vi "Test Runner Pre-build action.vi"(6 "Top Level/Always Included VIs":path[](array[path]), 7 "Main Destination Path":path, 9 "Target Name":string, 10 "Build Specification Name":string, 11 "Project Path":path) -> (0 "error out":errorcluster)   [LabVIEW 2013]
uses:
  classes/Test Runner/Test Runner.lvclass
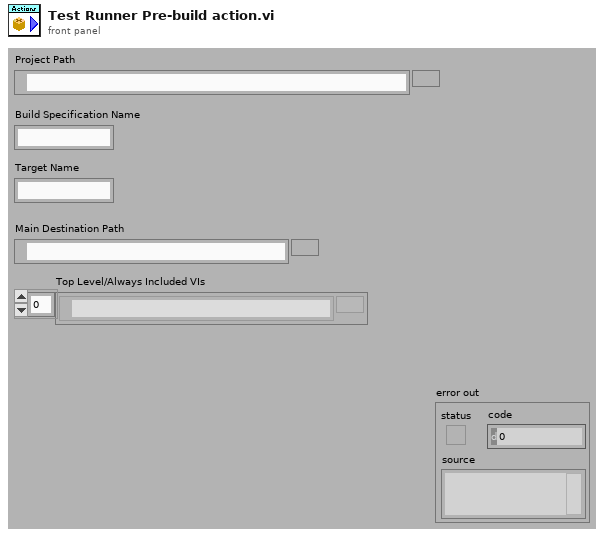
[diagram p1: front panel]
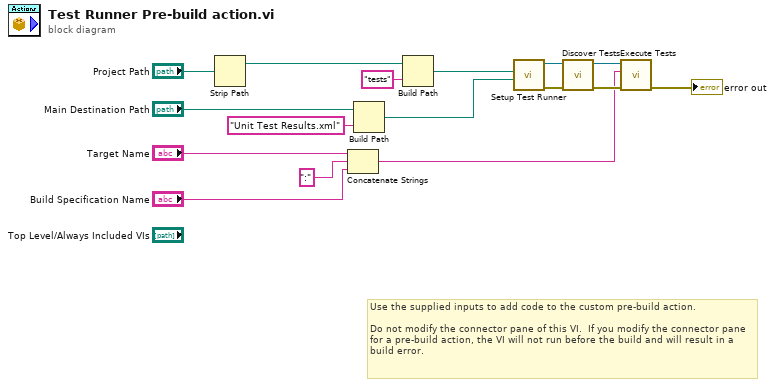
[diagram p0: block diagram]
diagram:
  # "Use the supplied inputs to add code to the custom pre-build action.\n\nDo not modify the connector pane of this VI.  If you modify the connector pane for a pre-build action, the VI will not run before the build and will result in a build error."
  n1 = Strip Path(path="Project Path") -> (stripped path=w1:path)  [unwired: 1 out]
  n2 = Concatenate Strings("Target Name", ":" ("string"), "Build Specification Name") -> (w6:string)
  n3 = Build Path(base path="Main Destination Path", name or relative path="Unit Test Results.xml") -> (appended path=w2:path)
  n4 = Build Path(base path=w1, name or relative path="tests") -> (appended path=w4:path)
  n5 = call "Setup Test Runner.vi"("Report Path"=w2, "Directory to search"=w4) -> ("error out"=w12:errorcluster, "Test Runner out"=w16:refnum<class "Test Runner.lvclass">)  [unwired: 8 in]
  n6 = call-dynamic "Discover Tests.vi"("error in (no error)"=w12, "Test Runner in"=w16) -> ("error out"=w10:errorcluster, "Test Runner out"=w11:refnum<class "Test Runner.lvclass">)  [unwired: 8 in]
  n7 = call-dynamic "Execute Tests.vi"("error in (no error)"=w10, "Suite Label"=w6, "Test Runner in"=w11) -> ("error out"=→"error out":errorcluster)  [unwired: 7 in, 1 out]
